vi "Get Pin Access.vi"(4 "Consumer Secret":string, 6 "Consumer Key":string, 7 "Signature Method":T1=enum."HMAC-SHA1", 8 "error in (no error)":errorcluster, 9 "Access URL":string, 10 "Authorize URL":string, 11 "Request URL":string) -> (0 "error out":errorcluster, 1 "body":string, 2 "headers":string, 3 "OAuth Credentials":T2={"Consumer Key"="", "Signature Method"=enum."HMAC-SHA1", "Token"="", "Version"="", "Token Secret"="", "Consumer Secret"=""})   [LabVIEW 2011, in "i3-oauth.lvlib"]
doc: "Obtains OAuth Credentials via PIN authorization for the application specified by the <B>Consumer Key</B> and <B>Consumer Secret</B>"
uses:
  i3-oauth.lvlib
  Controls/OAuth Credentials.ctl
  Controls/Signature Method.ctl
  <vilib>/Platform/browser.llb/Open URL in Default Browser (string).vi
panel:
  out "listening port":u16
  out "remote port":u16
  out "Post Data Transmitted":string
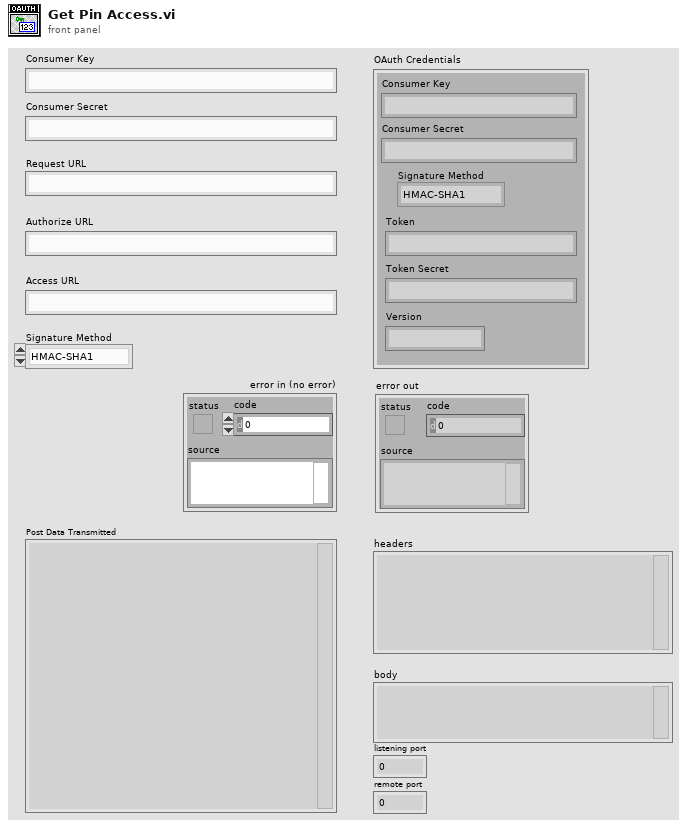
[diagram p1: front panel]
types:
  T1 = typedef "i3-oauth.lvlib/Signature Method.ctl" = enum16{"HMAC-MD5", "HMAC-SHA1", "HMAC-SHA224", "HMAC-SHA256", "HMAC-SHA384", "HMAC-SHA512"}
  T2 = typedef "i3-oauth.lvlib/OAuth Credentials.ctl" = cluster{"Consumer Key":string, "Signature Method":T1, "Token":string, "Version":string, "Token Secret":string, "Consumer Secret":string}
  T3 = enum16{"Standard", "Buffered", "CRLF", "Immediate"}
  T4 = typedef "i3-oauth.lvlib/key-value-pairs.ctl" = cluster{"key":string, "value":string}
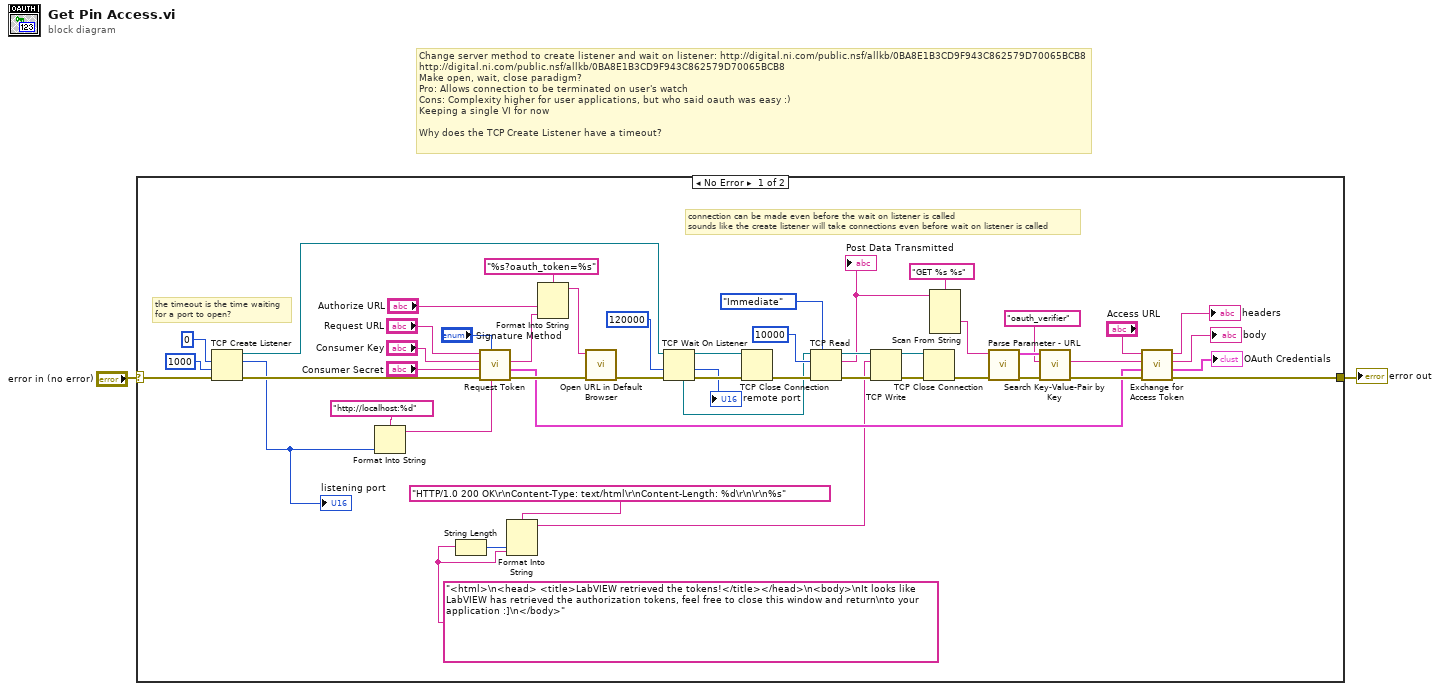
[diagram p0: block diagram]
diagram:
  # "Change server method to create listener and wait on listener: http://digital.ni.com/public.nsf/allkb/0BA8E1B3CD9F943C862579D70065BCB8\nhttp://digital.ni.com/public.nsf/allkb/0BA8E1B3CD9F943C862579D70065BCB8\nMake open, wait, close paradigm?\nPro: Allows connection to be terminated on user's watch\nCons: Complexity higher for user applications, but who said oauth was easy :)\nKeeping a single VI for now\n\nWhy does the TCP Create Listener have a timeout?"
  n1 = case shown="No Error" "error in (no error)" {
    selector: "error in (no error)" -> [w14 w52]
    tunnel: [w45 w52] -> w1
    frame No Error {
      w17 = "<html>\n<head> <title>LabVIEW retrieved the tokens!</title></head>\n<body>\nIt looks like LabVIEW has retrieved the authorization tokens, feel free to close this window and return\nto your application :]\n</body>"
      # "the timeout is the time waiting \nfor a port to open?"
      # "connection can be made even before the wait on listener is called\nsounds like the create listener will take connections even before wait on listener is called"
      n2 = TCP Create Listener(8:w14, 9:1000 ("timeout ms (25000)"), 10:u16 0 ("port")) -> (0:w15:errorcluster, 2:w11:u16, 3:w10:refnum<k5>)  [unwired: 2 in]
      "listening port" <- w11
      n3 = Format Into String(format string="http://localhost:%d" ("string"), w11) -> (resulting string=w38:string)  [unwired: 2 in, 1 out]
      n4 = String Length(string=w17) -> (length=w18:i32)
      n5 = call "Request Token.vi"("Callback URL"=w38, "Signature Method"="Signature Method", "error in (no error)"=w15, "Consumer Secret"="Consumer Secret", "Consumer Key"="Consumer Key", "Request URL"="Request URL") -> ("error out"=w51:errorcluster, "OAuth Credentials (request)"=w47:T2, "Request Token (duplicate)"=w30:string)  [unwired: 3 in]
      n6 = Format Into String(format string="HTTP/1.0 200 OK\r\nContent-Type: text/html\r\nContent-Length: %d\r\n\r\n%s" ("data in"), w18, w17) -> (resulting string=w16:string)  [unwired: 2 in, 1 out]
      n7 = Format Into String(format string="%s?oauth_token=%s", "Authorize URL", w30) -> (resulting string=w28:string)  [unwired: 2 in, 1 out]
      n8 = call-poly <vilib>:"Open URL in Default Browser.vi"("error in (no error)"=w51, "URL"=w28) -> ("error out"=w4:errorcluster)  [unwired: 4 in, 1 out]
      n9 = TCP Wait On Listener(8:w4, 9:120000 ("timeout ms (wait forever: -1)"), 11:w10) -> (0:w8:errorcluster, 1:→"remote port":u16, 3:w6:refnum<k5>, 4:w5:refnum<k5>)  [unwired: 1 in, 1 out]
      n10 = TCP Close Connection(connection ID=w6, error in (no error)=w8) -> (error out=w7:errorcluster)  [unwired: 1 in, 1 out]
      n11 = TCP Read(connection ID=w5, bytes to read=10000, error in (no error)=w7, 7:T3."Immediate" ("mode (standard)")) -> (connection ID out=w36:refnum<k5>, data out=w24:string, error out=w35:errorcluster)  [unwired: 1 in]
      "Post Data Transmitted" <- w24
      n12 = TCP Write(connection ID=w36, data in=w16, error in (no error)=w35) -> (connection ID out=w33:refnum<k5>, error out=w34:errorcluster)  [unwired: 1 in, 1 out]
      n13 = TCP Close Connection(connection ID=w33, error in (no error)=w34) -> (error out=w27:errorcluster)  [unwired: 1 in, 1 out]
      n14 = Scan From String(format string="GET %s %s", input string=w24) -> (output 1=w23:string)  [unwired: 5 in, 3 out]
      n15 = call "Parse Parameter - URL.vi"("error in (no error)"=w27, "URL"=w23) -> ("error out"=w26:errorcluster, "URL Parameters"=w22:T4[])  [unwired: 8 in]
      n16 = call "Search Key-Value-Pair by Key.vi"("error in (no error)"=w26, "Key"="oauth_verifier", "Key-Value-Pair List"=w22) -> ("error out"=w50:errorcluster, "Value"=w20:string)  [unwired: 6 in, 1 out]
      n17 = call "Exchange for Access Token.vi"("error in (no error)"=w50, "OAuth Credentials (request)"=w47, "Pin"=w20, "Access Request URL"="Access URL") -> ("error out"=w45:errorcluster, "OAuth Credentials (access)"=→"OAuth Credentials":T2, "body"=→"body":string, "headers"=→"headers":string)  [unwired: 4 in]
    }
    frame Error {
    }
  }
  "error out" <- w1
